vi "!2D-sample-tip-convolution.vi"() -> ()   [LabVIEW 2017]
panel:
  in  "Radius":dbl=10.0 min=-0.0 max=1000.0 format="%.2f"
  in  "Angle":dbl=20.0 min=1.0 max=89.0 format="%.2f"
  in  "Tip height":dbl=10.0 format="%#_13g"
  in  "Bias":dbl
  out "Intensity Graph 2":dbl[][](graph)
  out "Moving tip":dbl[][](graph)
  out "Sample Section":dynamicdata(graph)
  in  "Width X":dbl=157.0 format="%.2f"
  in  "Width Y":dbl=200.0 format="%.2f"
  in  "Period X":dbl=329.0 format="%.2f"
  in  "Spl Height":dbl=100.0 format="%.2f"
  in  "Period Y":dbl=333.0 format="%.2f"
  in  "Slope":dbl=41.0 format="%.2f"
  in  "index (row)":i32=150
  out "Intensity Graph":dbl[][](graph)
  in  "Pixels X":i32=500
  in  "Pixels Y":i32=500
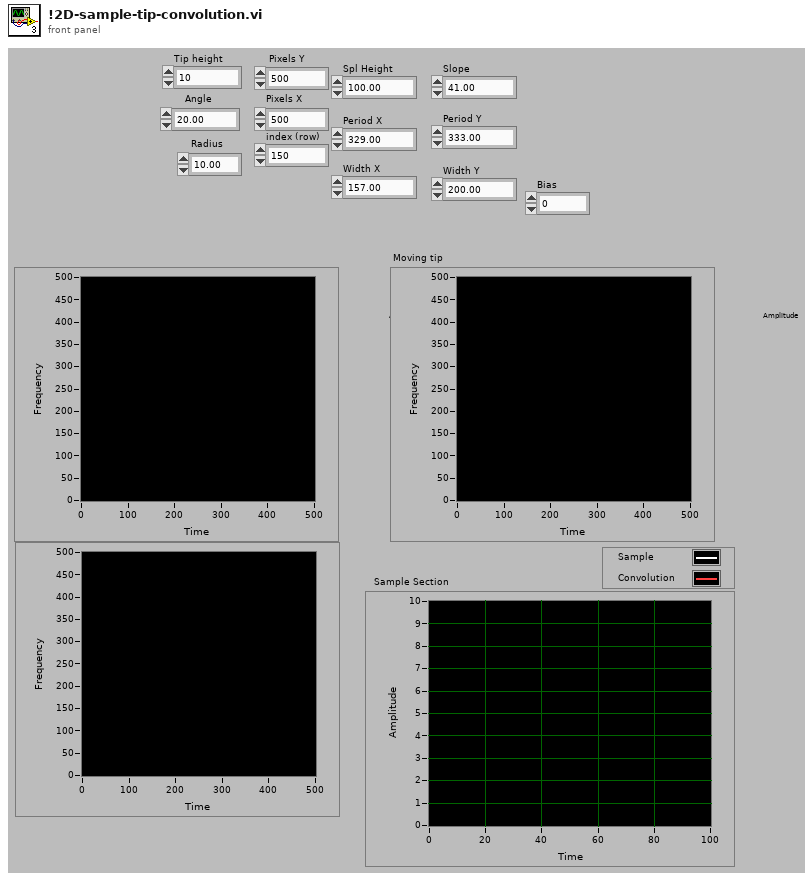
[diagram p1: front panel]
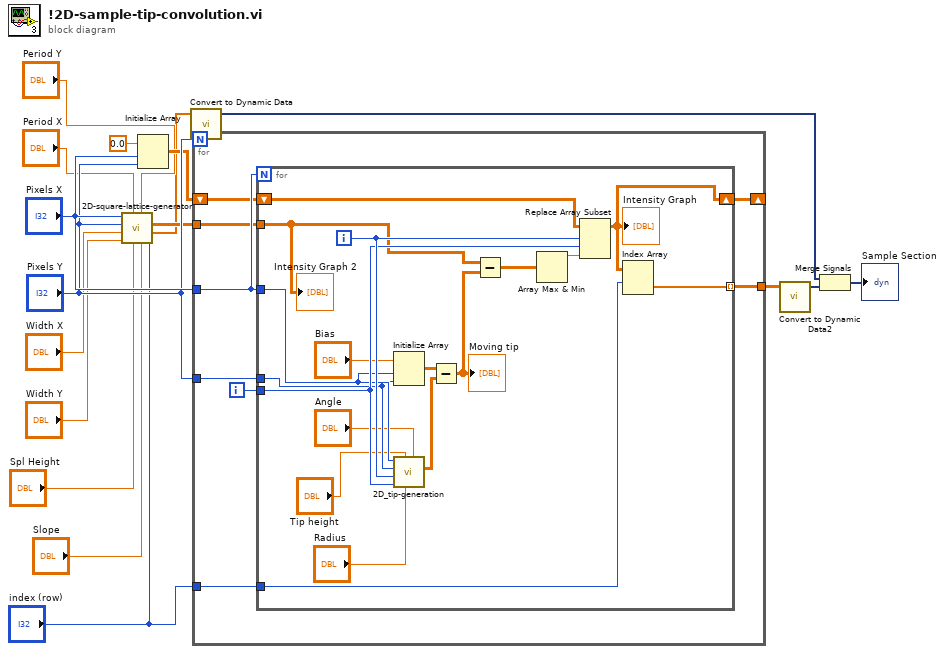
[diagram p0: block diagram]
diagram:
  n1 = call "2D-square-lattice-generator.vi"("index (row)"="index (row)", "Slope"="Slope", "Period Y"="Period Y", "Spl Height"="Spl Height", "Period X"="Period X", "Width Y"="Width Y", "Width X"="Width X", "Pixels Y"="Pixels Y", "Pixels X"="Pixels X") -> ("Sample Section"=w5:dbl[], "2D Sample"=w13:dbl[][])  [unwired: 1 in]
  n2 = Initialize Array(0.0 ("element"), "Pixels X", "Pixels Y") -> (w14:dbl[][])
  n3 = call "Convert to Dynamic Data"("Array"=w5) -> ("Dynamic Data Type"=w4:dynamicdata)  [unwired: 3 in]
  n4 = for {
    N: "Pixels Y" -> [_]
    tunnel: "Pixels Y" -> [w25]
    tunnel: "Pixels X" -> [w24]
    tunnel: w13 -> [w22]
    shift-right: [w20] -> _
    shift-left: w14 -> [w21]
    tunnel: "index (row)" -> [w19]
    tunnel: [w18] -> w3
    i -> [w23]
    n5 = for {
      N: w24 -> [_]
      tunnel: w25 -> [w36]
      tunnel: w24 -> [w37]
      tunnel: w23 -> [w40]
      tunnel: w22 -> [w39]
      shift-right: [w28] -> w20
      shift-left: w21 -> [w42]
      tunnel: w19 -> [w27]
      tunnel: [w26] -> w18 mode=indexing
      i -> [w41]
      n6 = Initialize Array("Bias", w37, w36) -> (w35:dbl[][])
      n7 = call "2D_tip-generation.vi"("Angle"="Angle", "Radius"="Radius", "Tip height"="Tip height", "Position Y"=w40, "Position X"=w41, "Pixels Y"=w36, "Pixels X"=w37) -> ("2D Tip"=w33:dbl[][])  [unwired: 3 in, 1 out]
      n8 = Subtract(x=w35, y=w33) -> (x-y=w34:dbl[][])
      "Moving tip" <- w34
      n9 = Subtract(x=w39, y=w34) -> (x-y=w43:dbl[][])
      n10 = Array Max & Min(array=w43) -> (max value=w38:dbl)  [unwired: 3 out]
      n11 = Replace Array Subset(array=w42, new element=w38, index (row)=w41, index (col)=w40) -> (w28:dbl[][])
      "Intensity Graph" <- w28
      n12 = Index Array(array=w28, index (row)=w27) -> (element=w26:dbl[])  [unwired: 1 in]
      "Intensity Graph 2" <- w39
    }
  }
  n13 = call "Convert to Dynamic Data2"("2D Array"=w3) -> ("Dynamic Data Type"=w2:dynamicdata)  [unwired: 3 in]
  n14 = Merge Signals(w4, w2) -> (→"Sample Section":dynamicdata)
